vi "Get ImageListRef.vi"(8 "error in (no error)":errorcluster caption="错误输入（无错误）", 11 "ImageListClass 输入":refnum<class "ImageListClass.lvclass"> caption="DNL_LabVIEW Object in") -> (0 "error out":errorcluster caption="错误输出", 2 "ImageList":refnum<k24>, 3 "ImageListClass 输出":refnum<class "ImageListClass.lvclass"> caption="DNL_LabVIEW Object out")   [LabVIEW 2013, in "ImageListClass.lvclass"]
uses:
  ImageListClass.lvclass
  System.Windows.Forms
  ImageListClass.lvclass/ImageListClass.ctl
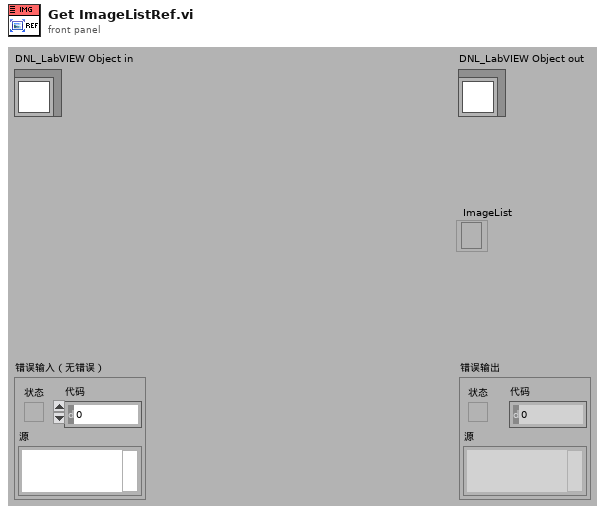
[diagram p1: front panel]
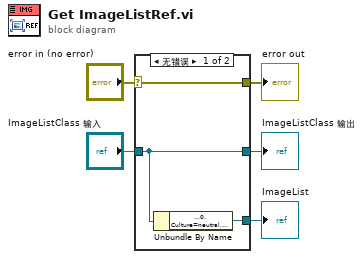
[diagram p0: block diagram]
diagram:
  n1 = case shown="无错误" "error in (no error)" {
    selector: "error in (no error)" -> [w8 w10]
    tunnel: [w8 w10] -> w4
    tunnel: [w7 w9] -> w2
    tunnel: "ImageListClass 输入" -> [w7 w9]
    tunnel: [w6 _] -> w1
    frame No Error {
      n2 = Unbundle By Name(w7) -> ("ImageList"=w6:refnum<k24>)
    }
    frame Error {
    }
  }
  "error out" <- w4
  "ImageListClass 输出" <- w2
  "ImageList" <- w1
